vi "To Variant.vi"(0 "Obj in":refnum<class "Termination.lvclass">, 11 "error in (no error)":errorcluster) -> (4 "Obj out":refnum<class "Termination.lvclass">, 8 "Array":variant[](array[variant]), 15 "error out":errorcluster)   [LabVIEW 2020, in "Termination.lvclass"]
uses:
  Termination.lvclass
  Termination.lvclass/Termination.ctl
  epl-vi-lib/Koop/KObject Class/KObject.lvclass
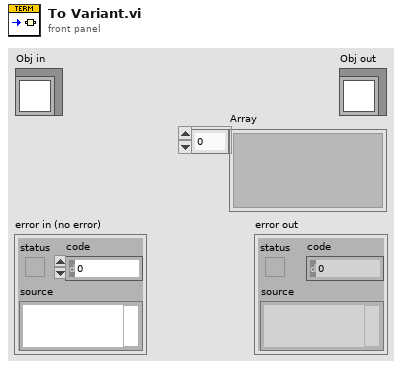
[diagram p1: front panel]
types:
  T1 = typedef "Termination.lvclass/Serialized.ctl" = cluster{"Type":T2, "Source":string, "Link to":string, "End after (ms)":dbl, "Latency (ms)":dbl, "Action":T3, "Nttl":i32, "Tttl":string, "one shot":bool, "TTL":refnum<class "TTLController.lvclass">[], "End on rep":bool, "Result":string, "Color":u32}
  T2 = typedef "Tosca-Event Type.ctl" = enum16{"Normal", "CS+", "CS-"}
  T3 = typedef "Tosca-Termination Condition Action.ctl" = enum16{"End state", "Complete state", "TTL only"}
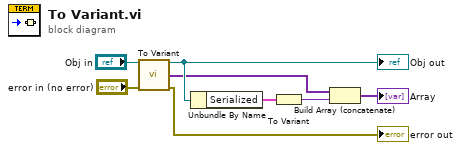
[diagram p0: block diagram]
diagram:
  n1 = call-parent "To Variant.vi"("KObject in"="Obj in", "error in (no error)"="error in (no error)") -> ("KObject out"=w3:refnum<class "Termination.lvclass">, "Array"=w2:variant[], "error out"=→"error out":errorcluster)  [unwired: 11 in]
  "Obj out" <- w3
  n2 = Unbundle By Name(w3) -> ("Serialized"=w4:T1)
  n3 = To Variant(anything=w4) -> (Variant=w5:variant)
  n4 = Build Array (concatenate)(w2, w5) -> (→"Array":variant[])
